vi "Spartan HTTP probe raw request.vi"(11 "Request":string) -> (3 "dup Request":string)   [LabVIEW 2011]
panel:
  in  "Backslash Codes?":bool
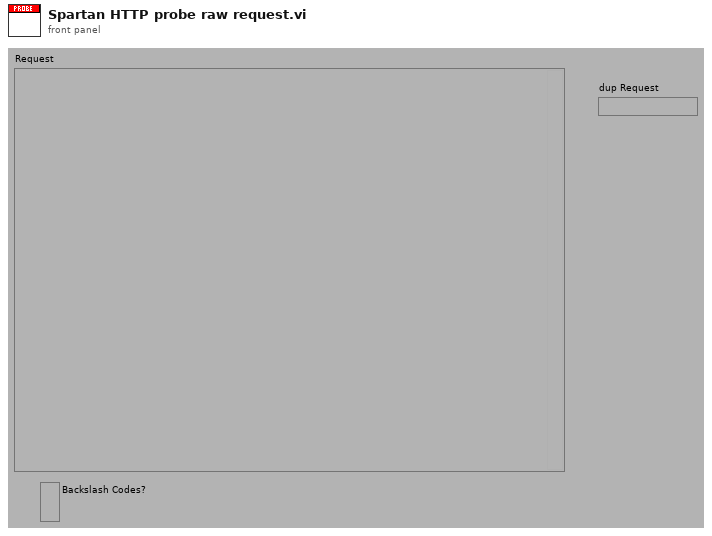
[diagram p1: front panel]
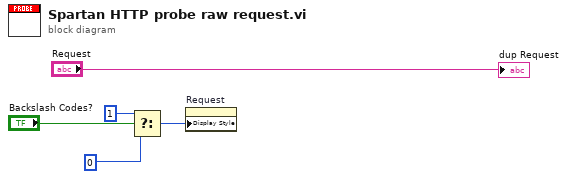
[diagram p0: block diagram]
diagram:
  n1 = Select(t=u32 1, s="Backslash Codes?", f=u32 0 ("Display Style")) -> (s? t:f=w4:u32)
  n2 = property on="Request" class="Str"("Display Style"=w4) -> ()  [unwired: 2 in, 2 out]
  "dup Request" <- "Request"
